vi "UIM Executable Build.vi"() -> ()   [LabVIEW 2015]
doc: "This example visualizes a way to specify plugins in code. This makes it easier to build executables that use the UIM API."
uses:
  Plugin UIPs/CaptionUIP/CaptionUIP.lvclass
  Plugin UIPs/DisabledUIP/DisabledUIP.lvclass
  Plugin UIPs/DescriptionUIP/DescriptionUIP.lvclass
  Plugin UIPs/PositionUIP/PositionUIP.lvclass
  Plugin UIPs/SizeUIP/SizeUIP.lvclass
  Plugin UIPs/TipStripUIP/TipStripUIP.lvclass
  Plugin UIPs/VisibleUIP/VisibleUIP.lvclass
  UIM/UIM.lvclass
panel:
  in  "Boolean":bool
  out "Waveform Chart":dbl(graph)
  in  "File Path Control":path
  in  "Numeric Control":dbl
  in  "String":string
  in  "Stop Button":bool
  in  "UI State":u16(ring) items=["English", "Polski"]
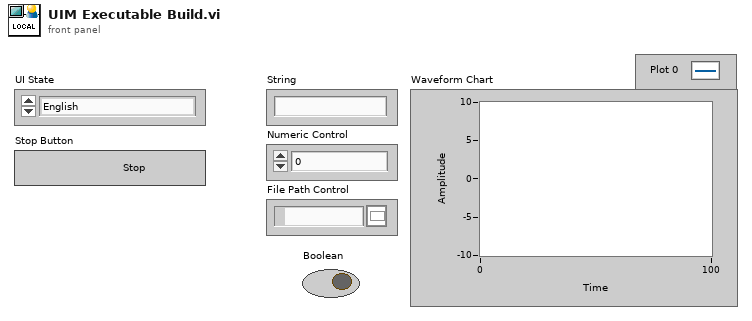
[diagram p1: front panel]
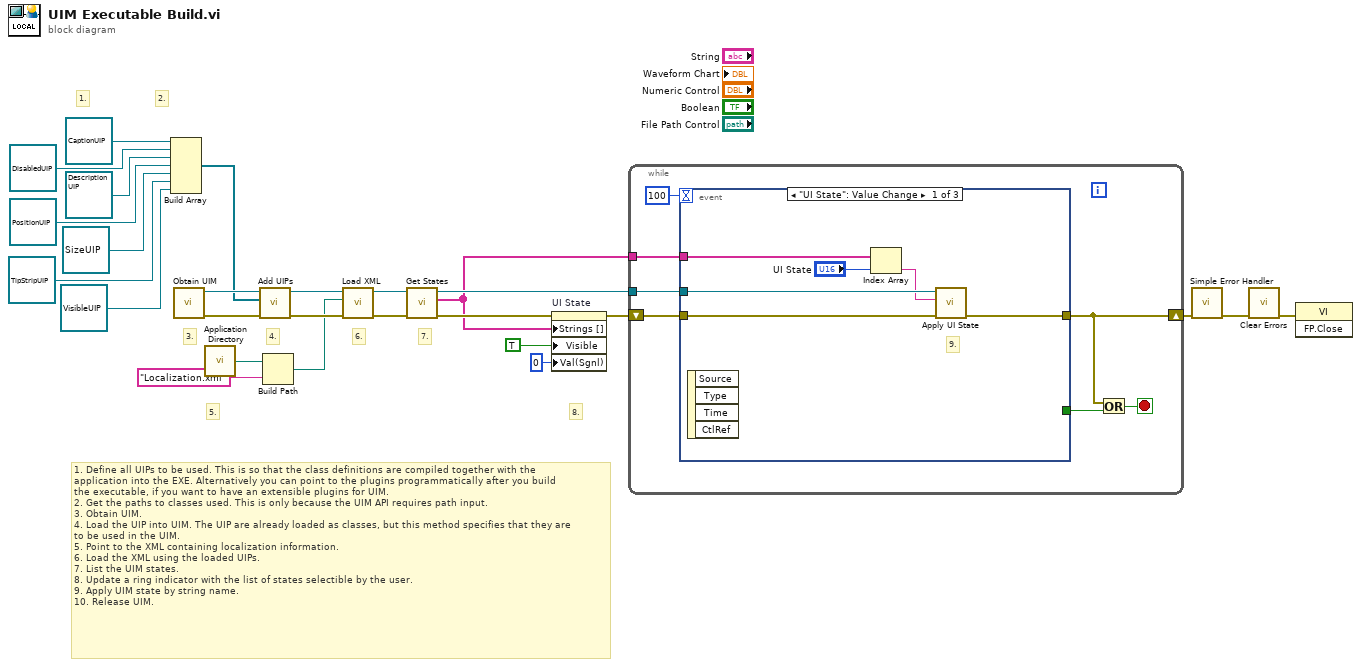
[diagram p0: block diagram]
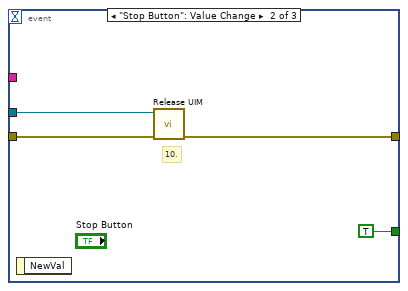
[diagram p2: hidden frame]
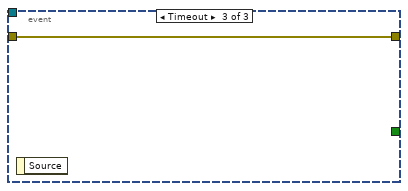
[diagram p3: hidden frame]
diagram:
  # "1. Define all UIPs to be used. This is so that the class definitions are compiled together with the\napplication into the EXE. Alternatively you can point to the plugins programmatically after you build\nthe executable, if you want to have an extensible plugins for UIM.\n2. Get the paths to classes used. This is only because the UIM API requires path input.\n3. Obtain UIM.\n4. Load the UIP into UIM. The UIP are already loaded as classes, but this method specifies that they are\nto be used in the UIM.\n5. Point to the XML containing localization information.\n6. Load the XML using the loaded UIPs.\n7. List the UIM states.\n8. Update a ring indicator with the list of states selectible by the user.\n9. Apply UIM state by string name.\n10. Release UIM."
  # "8."
  # "7."
  # "6."
  # "5."
  # "4."
  # "3."
  # "2."
  # "1."
  n1 = Build Array(refnum<class "CaptionUIP.lvclass"> refnum ("CaptionUIP.lvclass"), refnum<class "DisabledUIP.lvclass"> refnum ("DisabledUIP.lvclass"), refnum<class "DescriptionUIP.lvclass"> refnum ("DescriptionUIP.lvclass"), refnum<class "PositionUIP.lvclass"> refnum ("PositionUIP.lvclass"), refnum<class "SizeUIP.lvclass"> refnum ("SizeUIP.lvclass"), refnum<class "TipStripUIP.lvclass"> refnum ("TipStripUIP.lvclass"), refnum<class "VisibleUIP.lvclass"> refnum ("VisibleUIP.lvclass")) -> (w1:refnum<class "UIP.lvclass">[])
  n2 = call "Obtain UIM.vi"() -> ("Error Out"=w15:errorcluster, "UIM Handle"=w17:refnum<data-value>)  [unwired: 10 in]
  n3 = call <vilib>:"Application Directory.vi"() -> ("Application Directory"=w11:path)
  n4 = call "Add UIPs.vi"("Error In"=w15, "UIPs"=w1, "UIM In"=w17) -> ("Error Out"=w16:errorcluster, "UIM Out"=w14:refnum<data-value>)  [unwired: 7 in]
  n5 = Build Path(base path=w11, name or relative path="Localization.xml") -> (appended path=w12:path)
  n6 = call "Load XML.vi"("Error In"=w16, "XML File"=w12, "UIM In"=w14) -> ("Error Out"=w20:errorcluster, "UIM Out"=w23:refnum<data-value>)  [unwired: 7 in]
  n7 = call "Get States.vi"("Error In"=w20, "UIM In"=w23) -> ("Error Out"=w21:errorcluster, "States"=w19:string[], "UIM Out"=w22:refnum<data-value>)  [unwired: 7 in]
  n8 = property on="UI State" class="Ring (strict)"(error in=w21, "Strings []"=w19, "Visible"=TRUE, "Val(Sgnl)"=u16 0 ("Value (Signaling)")) -> (error out=w26:errorcluster)  [unwired: 1 in, 1 out]
  n9 = while {
    tunnel: w22 -> [w33]
    tunnel: w19 -> [w31]
    shift-right: [w28] -> w18
    shift-left: w26 -> [w32]
    stop <- w29 stop-if-true
    n10 = event shown="[0] \"UI State\": Value Change" {
      selector: _ -> [_ _ _]
      dyn-events: _ -> [_ _ _]
      timeout: 100 -> [_ _ _]
      tunnel: w33 -> [w39 w42 _]
      tunnel: [_ TRUE _] -> w30
      tunnel: w32 -> [w38 w41 w44]
      tunnel: [w37 w40 w44] -> w28
      tunnel: w31 -> [w34 _ _]
      event "UI State": Value Change {
        # "9."
        n11 = event-data() -> ()  [unwired: 1 in, 4 out]
        n12 = Index Array(array=w34, index="UI State") -> (element=w35:string)
        n13 = call "Apply UI State.vi"("Error In"=w38, "State Name"=w35, "UIM In"=w39) -> ("Error Out"=w37:errorcluster)  [unwired: 7 in, 1 out]
      }
      event "Stop Button": Value Change {
        # "10."
        n14 = event-data() -> ()  [unwired: 1 in, 1 out]
        n15 = call "Release UIM.vi"("Error In"=w41, "UIM Handle"=w42) -> ("Error Out"=w40:errorcluster)  [unwired: 9 in]
      }
      event Timeout {
        n16 = event-data() -> ()  [unwired: 1 in, 1 out]
      }
    }
    n17 = Or(x=w28, y=w30) -> (x .or. y?=w29:bool)
  }
  n18 = call <vilib>:"Simple Error Handler.vi"("error in (no error)"=w18) -> ("error out"=w3:errorcluster)  [unwired: 4 in, 4 out]
  n19 = call <vilib>:"Clear Errors.vi"("error in (no error)"=w3) -> ("error out"=w2:errorcluster)  [unwired: 5 in, 1 out]
  n20 = invoke class="VI" method="FP.Close"(error in=w2) -> ()  [unwired: 2 in, 3 out]
